vi "transform.vi"(9 "?":bool, 11 "x*y":waveform(dbl)) -> (3 "Power Spectrum":cluster{"f0":dbl, "df":dbl, "magnitude":dbl[]})   [LabVIEW 2024]
uses:
  <vilib>/Analysis/baseanly.llb/Mean (DBL).vi
  <vilib>/express/express analysis/Spectral/Block/exnSpectralBlock spectral measurements power poly.vi
  <vilib>/express/express analysis/Spectral/Block/exnSpectralBlock spectral measurements power WFM.vi
  <vilib>/express/express analysis/Spectral/XNode/ExpressSpectralMeasurementsBlockNode.xnode
  <vilib>/Analysis/NI_AALBase.lvlib
  <vilib>/Analysis/NI_AALPro.lvlib
  <vilib>/measure/NI_MAPro.lvlib
  <vilib>/measure/maspectr.llb/FFT Spectrum (Mag-Phase) for 1 Chan.vi
panel:
  in  "dB On (F)":bool
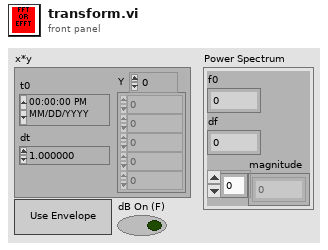
[diagram p1: front panel]
types:
  T1 = cluster{"averaging mode":u16, "weighting mode":u16, "number of averages":u32}
  T2 = cluster{"dB On (F)":bool, "unwrap phase (F)":bool, "convert to degree (F)":bool}
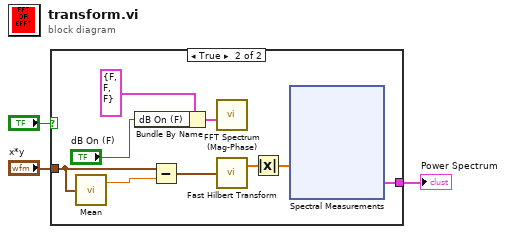
[diagram p0: block diagram]
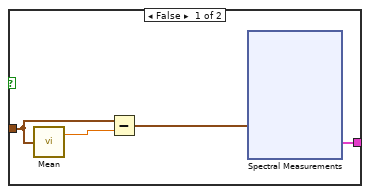
[diagram p2: hidden frame]
diagram:
  n1 = case shown="True" "?" {
    tunnel: "x*y" -> [w6 w24]
    tunnel: [w4 w20] -> w2
    frame False {
      n2 = call-poly <vilib>:"Mean.vi"("X"=w6) -> ("mean"=w7:dbl)  [unwired: 1 out]
      n3 = Subtract(x=w6, y=w7) -> (x-y=w5:waveform(dbl))
      n4 = xnode "Spectral Measurements"("Signals"=w5) -> ("Power Spectrum"=w4:cluster{"f0":dbl, "df":dbl, "magnitude":dbl[]})  [unwired: 1 in, 1 out]
    }
    frame True {
      n5 = call-poly <vilib>:"Mean.vi"("X"=w24) -> ("mean"=w25:dbl)  [unwired: 1 out]
      n6 = Bundle By Name(cluster=T2 {"dB On (F)"=FALSE, "unwrap phase (F)"=FALSE, "convert to degree (F)"=FALSE} ("view"), "dB On (F)"="dB On (F)") -> (w17:T2)
      n7 = Subtract(x=w24, y=w25) -> (x-y=w23:waveform(dbl))
      n8 = call-poly <vilib>:"FFT Spectrum (Mag-Phase).vi"("view"=w17) -> ()  [unwired: 6 in, 5 out]
      n9 = call <vilib>:"Fast Hilbert Transform.vi"("X"=w23) -> ("Hilbert{X}"=w22:dbl[])  [unwired: 1 out]
      n10 = Absolute Value(x=w22) -> (abs(x)=w21:dbl[])
      n11 = xnode "Spectral Measurements"("Signals"=w21) -> ("Power Spectrum"=w20:cluster{"f0":dbl, "df":dbl, "magnitude":dbl[]})  [unwired: 1 in, 1 out]
    }
  }
  "Power Spectrum" <- w2
